vi "DFD Integer Delay (Wfm).vi"(7 "init? (F)":bool, 8 "error in (no error)":errorcluster, 10 "delay":i32, 11 "signal in":waveform(dbl)={"t0"=timestamp(0 s since 1904-01-01), "dt"=0.0, "Y"=[]}) -> (0 "error out":errorcluster, 3 "signal out":waveform(dbl))   [LabVIEW 2017, in "NI_DigFilterLicensed.lvlib"]
doc: "Delays a signal continuously by a specified integer number of sample intervals. Wire data to the <B>signal in</B> input to determine the polymorphic instance to use or manually select the instance."
uses:
  <vilib>/addons/Digital Filter Design/NI_DigFilterLicensed.lvlib
  <vilib>/addons/Digital Filter Design/Process.llb/DFD Integer Delay with State (Array).vi
  <vilib>/addons/Digital Filter Design/NI_DigFilter_Process.lvlib
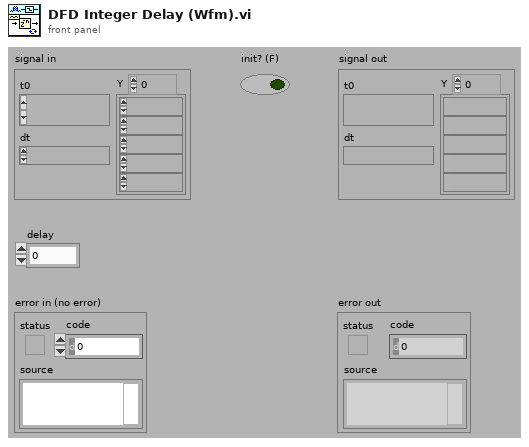
[diagram p1: front panel]
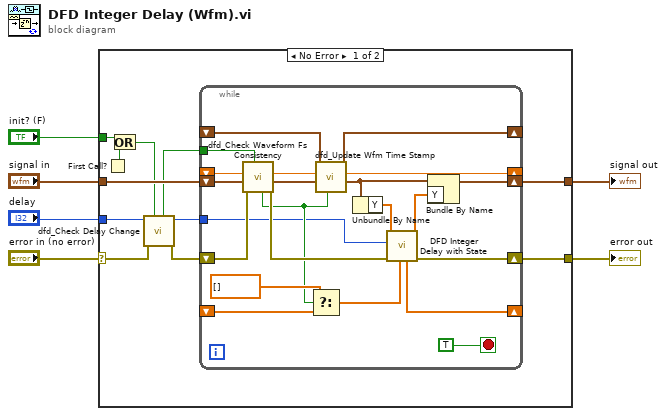
[diagram p0: block diagram]
diagram:
  n1 = case shown="No Error" "error in (no error)" {
    selector: "error in (no error)" -> [w8 w39]
    tunnel: [w15 w39] -> w5
    tunnel: "signal in" -> [w17 _]
    tunnel: [w16 _] -> w3
    tunnel: "delay" -> [w12 _]
    tunnel: "init? (F)" -> [w13 _]
    frame No Error {
      n2 = First Call?() -> (First Call?: T/F=w14:bool)
      n3 = Or(x=w13, y=w14) -> (x .or. y?=w10:bool)
      n4 = call <vilib>:"dfd_Check Delay Change.vi"("init in"=w10, "error in (no error)"=w8, "delay in"=w12) -> ("error out"=w7:errorcluster, "delay out"=w11:i32, "init out"=w9:bool)  [unwired: 6 out]
      n5 = while {
        shift-right: [w37] -> _
        shift-left: _ -> [w36]
        shift-right: [w31] -> _
        shift-left: _ -> [w32]
        tunnel: w11 -> [w18]
        shift-right: [w22] -> w16
        shift-left: w17 -> [w33]
        shift-right: [w20] -> w15
        shift-left: w7 -> [w26]
        shift-right: [w27] -> _
        shift-left: _ -> [w28]
        tunnel: w9 -> [w30]
        stop <- TRUE stop-if-true
        n6 = call <vilib>:"dfd_Check Waveform Fs Consistency.vi"("init in"=w30, "error in (no error)"=w26, "signal in"=w33, "dt in"=w32) -> ("error out"=w25:errorcluster, "signal out"=w29:waveform(dbl), "dt out"=w31:dbl, "init out"=w19:bool)  [unwired: 4 out]
        n7 = Select(t=dbl[] [], s=w19, f=w36) -> (s? t:f=w35:dbl[])
        n8 = call <vilib>:"dfd_Update Wfm Time Stamp.vi"("init? (F)"=w19, "signal in"=w29, "t0"=w28) -> ("signal out"=w23:waveform(dbl), "tf"=w27:timestamp)  [unwired: 7 out]
        n9 = Unbundle By Name(w23) -> ("Y"=w24:dbl[])
        n10 = call-poly <vilib>:"DFD Integer Delay with State.vi"("state in"=w35, "error in (no error)"=w25, "delay"=w18, "signal in"=w24) -> ("error out"=w20:errorcluster, "signal out"=w21:dbl[], "state out"=w37:dbl[])  [unwired: 5 out]
        n11 = Bundle By Name(cluster=w23, "Y"=w21) -> (w22:waveform(dbl))
      }
    }
    frame Error {
    }
  }
  "error out" <- w5
  "signal out" <- w3
